vi "Abort.vi"(8 "error in (no error)":errorcluster, 11 "Execution API in":refnum<class "Execution API.lvclass">) -> (0 "error out":errorcluster, 3 "Execution API out":refnum<class "Execution API.lvclass">)   [LabVIEW 2020, in "Execution API.lvclass"]
doc: "Aborts a running execution."
uses:
  Execution API.lvclass
  Execution API.lvclass/Execution API.ctl
  Test Runner/Test Runner.lvclass/Test Runner.ctl
  Test Runner/Test Runner.lvclass
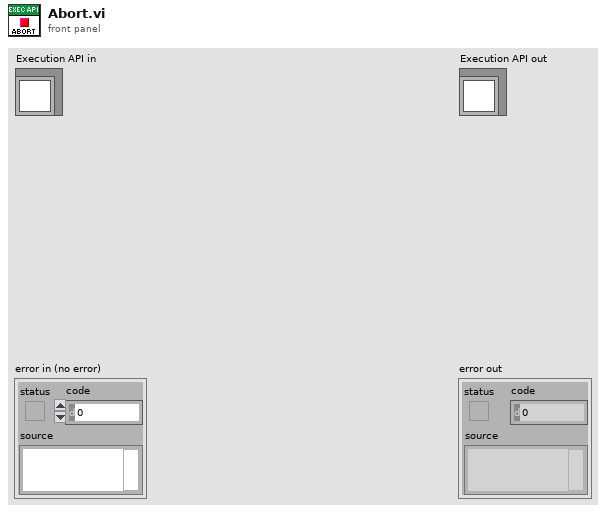
[diagram p1: front panel]
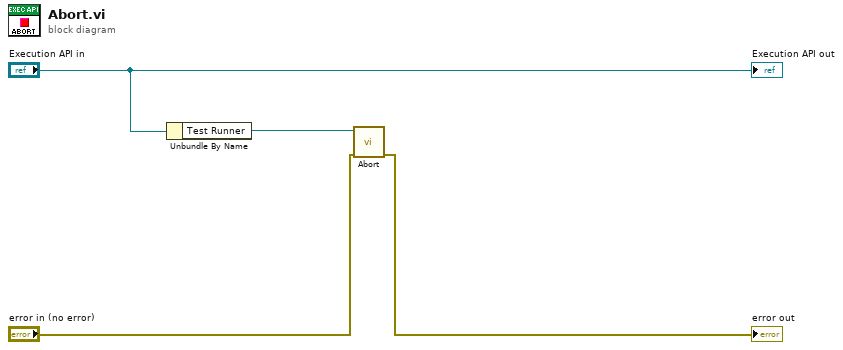
[diagram p0: block diagram]
diagram:
  n1 = Unbundle By Name("Execution API in") -> ("Test Runner"=w3:refnum<class "Test Runner.lvclass">)
  n2 = call "Abort.vi"("error in (no error)"="error in (no error)", "Test Runner In"=w3) -> ("error out"=→"error out":errorcluster)  [unwired: 8 in, 1 out]
  "Execution API out" <- "Execution API in"
